vi "DTbl Empty Digital.vi"() -> (1 "digital data":digitaldata)   [LabVIEW 2018]
doc: "Returns empty digital data. Use this constant to initialize shift registers or build digital tables."
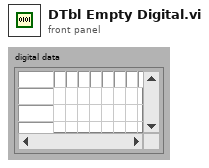
[diagram p1: front panel]
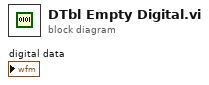
[diagram p0: block diagram]
diagram:
